vi "sync init all semaphores.vi"(8 "error in (no error)":errorcluster, 10 "pointer to shared memory":u64, 11 "sync items":T3[](array[typedef])) -> (0 "error out":errorcluster, 2 "offset pointer out":u64, 3 "initialized semaphores":T1[](array[typedef]))   [LabVIEW 2013, in "Shared Memory runtime.lvclass"]
uses:
  Shared Memory runtime.lvclass
  editor node/sync/sync item.ctl
  editor node/sync/sync mechanism.ctl
  controls/semaphore data.ctl
  <vilib>/NI/Pthreads for LabVIEW on Linux RT/Classes/Semaphore/Controls/reference.ctl
  <vilib>/NI/Pthreads for LabVIEW on Linux RT/Classes/Semaphore/Semaphore.lvclass
  configuration/Shared Memory configuration.lvclass
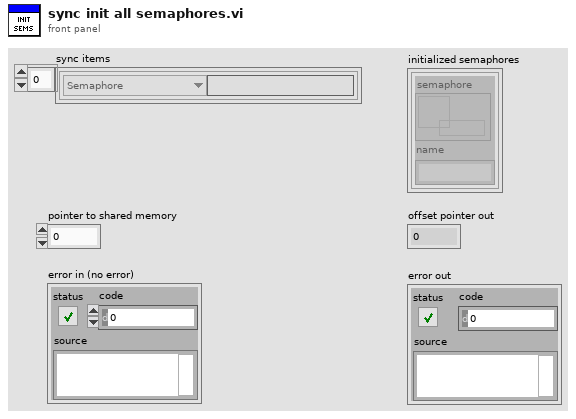
[diagram p1: front panel]
types:
  T1 = typedef "Shared Memory runtime.lvclass/semaphore data.ctl" = cluster{"semaphore":T2, "name":string}
  T2 = typedef "POSIX Threads.lvlib/Semaphore.lvclass/reference.ctl" = refnum<data-value>
  T3 = typedef "Shared Memory configuration.lvclass/sync item.ctl" = cluster{"mechanism":T4, "name":string}
  T4 = typedef "Shared Memory configuration.lvclass/sync mechanism.ctl" = enum16{"Semaphore", "Conditional Variable"}
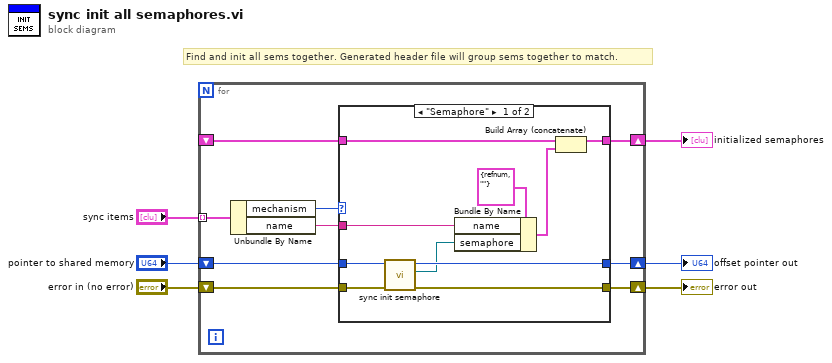
[diagram p0: block diagram]
diagram:
  # "Find and init all sems together. Generated header file will group sems together to match."
  n1 = for {
    tunnel: "sync items" -> [w15] mode=indexing
    shift-right: [w14] -> w3
    shift-left: _ -> [w13]
    shift-right: [w8] -> w2
    shift-left: "pointer to shared memory" -> [w9]
    shift-right: [w7] -> w1
    shift-left: "error in (no error)" -> [w10]
    n2 = Unbundle By Name(w15) -> ("mechanism"=w12:T4, "name"=w11:string)
    n3 = case shown="\"Semaphore\"" w12 {
      tunnel: [w23 w28] -> w14
      tunnel: w13 -> [w22 w28]
      tunnel: w11 -> [w18 _]
      tunnel: w10 -> [w21 w27]
      tunnel: w9 -> [w20 w26]
      tunnel: [w19 w26] -> w8
      tunnel: [w16 w27] -> w7
      frame "Semaphore" {
        n4 = call "sync init semaphore.vi"("error in (no error)"=w21, "pointer in"=w20) -> ("error out"=w16:errorcluster, "Semaphore out"=w17:T2, "offset pointer out"=w19:u64)  [unwired: 7 in]
        n5 = Bundle By Name(cluster=T1 {"semaphore"=refnum, "name"=""} ("semaphore data"), "name"=w18, "semaphore"=w17) -> (w24:T1)
        n6 = Build Array (concatenate)(w22, w24) -> (w23:T1[])
      }
      frame Default {
      }
    }
  }
  "initialized semaphores" <- w3
  "offset pointer out" <- w2
  "error out" <- w1
